vi "downsample.vi"(8 "error in (no error)":errorcluster, 9 "y factor":dbl=1.0 min=1.0, 10 "x factor":dbl=1.0 min=1.0, 11 "Image in":refnum<class "Image.lvclass">) -> (0 "error out":errorcluster, 3 "Image out":refnum<class "Image.lvclass">)   [LabVIEW 2010, in "Image.lvclass"]
uses:
  Image.lvclass
  storage_mode.ctl
  ErrorController/ErrorController/class_data.vi
  <vilib>/vision/NI_Vision_Development_Module.lvlib
  ErrorController/ErrorController/ErrorController.lvclass
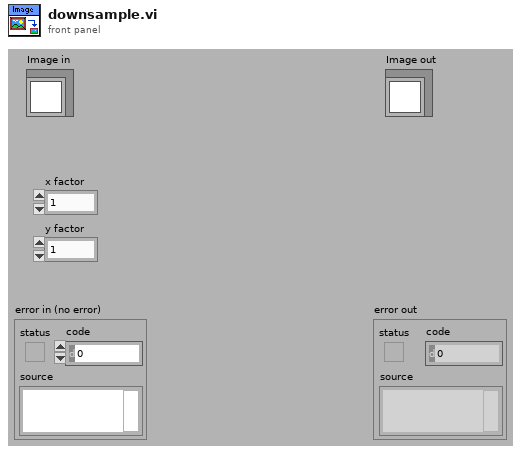
[diagram p1: front panel]
types:
  T1 = typedef "Image.lvclass/storage_mode.ctl" = enum16{"RAM", "disk"}
  T2 = typedef "Image Type" = u32
  T3 = typedef "IMAQ Image.ctl" = refnum<image>
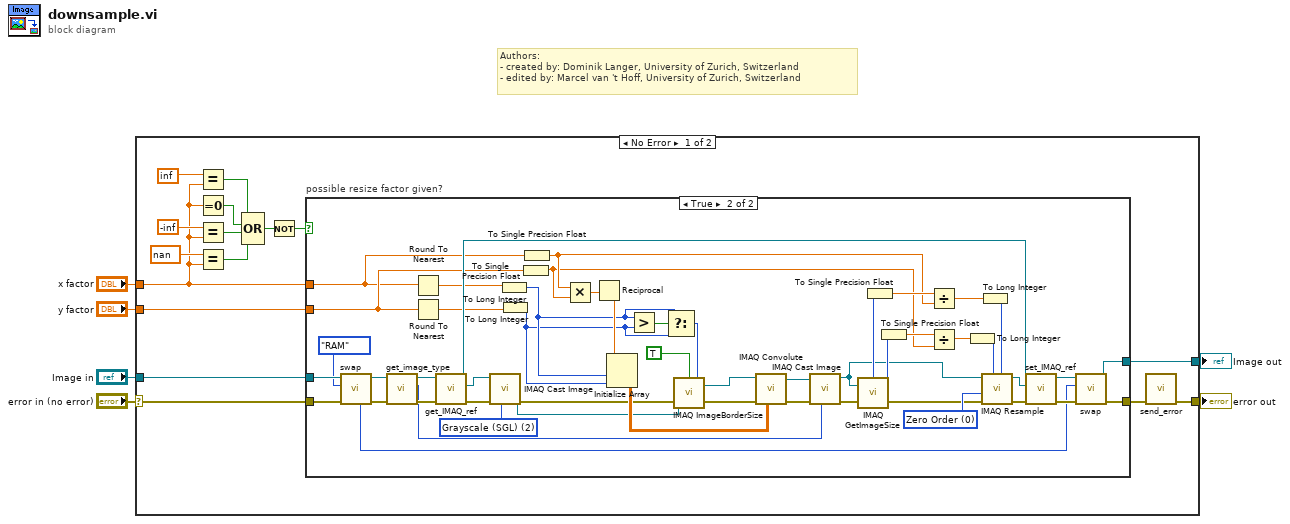
[diagram p0: block diagram]
diagram:
  # "Authors: \n- created by: Dominik Langer, University of Zurich, Switzerland\n- edited by: Marcel van 't Hoff, University of Zurich, Switzerland"
  n1 = case shown="No Error" "error in (no error)" {
    selector: "error in (no error)" -> [w21 w77]
    tunnel: [w8 w77] -> w5
    tunnel: [w22 w76] -> w3
    tunnel: "Image in" -> [w20 w76]
    tunnel: "x factor" -> [w15 _]
    tunnel: "y factor" -> [w19 _]
    frame No Error {
      n2 = Equal?(x=inf, y=w15) -> (x = y?=w14:bool)
      n3 = Equal To 0?(x=w15) -> (x = 0?=w13:bool)
      n4 = Equal?(x=-inf, y=w15) -> (x = y?=w12:bool)
      n5 = Equal?(x=nan, y=w15) -> (x = y?=w11:bool)
      n6 = Compound Arithmetic op=OR(w14, w13, w12, w11) -> (w10:bool)
      n7 = Not(x=w10) -> (.not. x?=w9:bool)
      n8 = case "possible resize factor given?" shown="True" w9 {
        tunnel: [w24 w61] -> w7
        tunnel: [w23 w59] -> w22
        tunnel: w21 -> [w24 w57]
        tunnel: w20 -> [w23 w56]
        tunnel: w19 -> [_ w39]
        tunnel: w15 -> [_ w25]
        frame False {
        }
        frame True {
          w47 = T2 2 items=["Grayscale (U8)", "Grayscale (I16)", "Grayscale (SGL)", "Complex (CSG)", "RGB (U32)", "HSL (U32)", "RGB (U64)", "Grayscale (U16)"] ("Image Type")
          w75 = u32 0 items=["Zero Order", "Bi-Linear", "Quadratic", "Cubic Spline"] ("Interpolation Type")
          n9 = call-dynamic "swap.vi"("error in (no error)"=w57, "storage type target"=storage_mode."RAM", "Image in"=w56) -> ("error out"=w51:errorcluster, "Image out"=w50:refnum<class "Image.lvclass">, "previous storage mode"=w55:T1)  [unwired: 6 out]
          n10 = call-dynamic "get_image_type.vi"("error in (no error)"=w51, "Image.lvclass in"=w50) -> ("error out"=w49:errorcluster, "Image Type"=w43:T2, "Image.lvclass out"=w48:refnum<class "Image.lvclass">)  [unwired: 7 out]
          n11 = Round To Nearest(number=w25) -> (nearest integer value=w41:dbl)
          n12 = Round To Nearest(number=w39) -> (nearest integer value=w42:dbl)
          n13 = call-dynamic "get_IMAQ_ref.vi"("error in (no error)"=w49, "Image.lvclass in"=w48) -> ("error out"=w53:errorcluster, "Image"=w52:T3, "Image.lvclass out"=w58:refnum<class "Image.lvclass">)  [unwired: 7 out]
          n14 = call "IMAQ Cast Image"("Image Type"=w47, "error in (no error)"=w53, "Image Src"=w52) -> ("error out"=w32:errorcluster, "Image Dst Out"=w28:T3)  [unwired: 3 in, 4 out]
          n15 = To Long Integer(number=w41) -> (32bit integer=w34:i32)
          n16 = To Long Integer(number=w42) -> (32bit integer=w33:i32)
          n17 = To Single Precision Float(number=w39) -> (single precision float=w37:sgl)
          n18 = To Single Precision Float(number=w25) -> (single precision float=w38:sgl)
          n19 = Multiply(x=w38, y=w37) -> (x*y=w40:sgl)
          n20 = Reciprocal(x=w40) -> (1/x=w65:sgl)
          n21 = Initialize Array(w65, w34, w33) -> (w36:sgl[][])
          n22 = Greater?(x=w34, y=w33) -> (0:w35:bool)
          n23 = Select(t=w34, s=w35, f=w33) -> (s? t:f=w29:i32)
          n24 = call "IMAQ ImageBorderSize"("Get/Set Status? (Set)"=TRUE, "Image"=w28, "Image border size in"=w29, "error in (no error)"=w32) -> ("Image Out"=w27:T3, "error out"=w31:errorcluster)  [unwired: 1 out]
          n25 = call "IMAQ Convolute"("Kernel"=w36, "error in (no error)"=w31, "Image Src"=w27) -> ("error out"=w30:errorcluster, "Image Dst Out"=w46:T3)  [unwired: 4 in, 3 out]
          n26 = call "IMAQ Cast Image"("Image Type"=w43, "error in (no error)"=w30, "Image Src"=w46) -> ("error out"=w45:errorcluster, "Image Dst Out"=w44:T3)  [unwired: 3 in, 4 out]
          n27 = call "IMAQ GetImageSize"("Image"=w44, "error in (no error)"=w45) -> ("Y Resolution"=w68:i32, "X Resolution"=w67:i32, "error out"=w66:errorcluster)  [unwired: 2 out]
          n28 = To Single Precision Float(number=w67) -> (single precision float=w69:sgl)
          n29 = To Single Precision Float(number=w68) -> (single precision float=w70:sgl)
          n30 = Divide(x=w69, y=w38) -> (x/y=w71:sgl)
          n31 = Divide(x=w70, y=w37) -> (x/y=w72:sgl)
          n32 = To Long Integer(number=w72) -> (32bit integer=w73:i32)
          n33 = To Long Integer(number=w71) -> (32bit integer=w74:i32)
          n34 = call "IMAQ Resample"("X Resolution"=w74, "Y Resolution"=w73, "error in (no error)"=w66, "Interpolation Type"=w75, "Image Src"=w44) -> ("error out"=w64:errorcluster, "Image Dst Out"=w63:T3)  [unwired: 2 in, 3 out]
          n35 = call-dynamic "set_IMAQ_ref.vi"("error in (no error)"=w64, "Image"=w63, "Image.lvclass in"=w58) -> ("error out"=w62:errorcluster, "Image.lvclass out"=w60:refnum<class "Image.lvclass">)  [unwired: 7 out]
          n36 = call-dynamic "swap.vi"("error in (no error)"=w62, "storage type target"=w55, "Image in"=w60) -> ("error out"=w61:errorcluster, "Image out"=w59:refnum<class "Image.lvclass">)  [unwired: 7 out]
        }
      }
      n37 = call "send_error.vi"("error in (no error)"=w7) -> ("error out"=w8:errorcluster)  [unwired: 10 in]
    }
    frame Error {
    }
  }
  "error out" <- w5
  "Image out" <- w3
